vi "DAQ_pp3c_AudioRetrigger.vi"(0 "Daq config In":T6={"Sound AO"="Dev6/ao0", "Shock intesity AO"="Dev6/ao1", "Code_LED DO"="Dev6/port1:2", "Switch DI"="Dev6/port1/line0", "Webcam"="cam9", "Sound AO task"="", "Sound card task"=0, "Shock intensity AO task"="", "Code_LED DO task"="", "Switch DI task"="", "AO <=> Sound card"=FALSE, "Sound card"=0, "sample rate"=100000.0, "Variable shock"=TRUE, "Webcam on"=FALSE, "Waveform memo"={"t0"=timestamp(0 s since 1904-01-01), "dt"=1.0, "Y"=[]}, "Tone trigger"="PFI1", "Master-9 DO"="", "Master-9 DO task"="Dev6/port0/line5:7"} {"sample rate" min=8000.0; "Sound card task" format="%.0x"}, 5 "State In":T1={"Curr  tr"=0, "Curr (ms)"=0, "Cum (ms)"=0, "Run loop diff"=0, "Tone countdown (ms)"=0, "Countdown (ms)"=0, "Curr State"=enum."0 NULL", "Prev State"=enum."1 Habituation", "Rw"=FALSE, "Sw"=FALSE, "Tone\nGate"=FALSE, "Punish"=FALSE, "Current DAQ DO Int"=0, "Current Loaded Trial"={"Trial Type Number"=1, "Trial Type"=enum."GO", "Trial Weight"=100, "Shock (mA)"=0.3, "Duration (ms)"=0.25, "Sound Type"=enum."04 FM Sweep", "Stim P1"=4000.0, "Stim P2"=0.0, "Stim P3"=0.0, "Stim P4"=2000.0, "DAQ Amplitude (V)"=0.25}, "Next Trial (for display purposes)"={"Trial Type Number"=1, "Trial Type"=enum."GO", "Trial Weight"=100, "Shock (mA)"=0.3, "Duration (ms)"=0.25, "Sound Type"=enum."04 FM Sweep", "Stim P1"=4000.0, "Stim P2"=0.0, "Stim P3"=0.0, "Stim P4"=2000.0, "DAQ Amplitude (V)"=0.25}, "Total trials memo"=0, "State start cum memo (ms)"=0, "Last dur jump time memo (ms)"=0, "Last dur shock time memo (ms)"=0, "Tone repeat memo (ms)"=0, "Webcam on"=FALSE, "Webcam recording"=FALSE, "State update flag"=FALSE, "Last loaded shock voltage"=0.0, "Vid upd"=enum."0"} {"Current DAQ DO Int" format="%016b"; "Next Trial (for display purposes)"."DAQ Amplitude (V)" min=0.0 max=5.0 format="%_4g"; "Next Trial (for display purposes)"."Shock (mA)" min=-1.0 max=5.0; "Next Trial (for display purposes)"."Trial Weight" step=1; "Next Trial (for display purposes)"."Duration (ms)" min=0.0 max=1.0; "Next Trial (for display purposes)"."Trial Type Number" min=1 max=256 step=1; "Current Loaded Trial"."DAQ Amplitude (V)" min=0.0 max=5.0 format="%_4g"; "Current Loaded Trial"."Shock (mA)" min=-1.0 max=5.0; "Current Loaded Trial"."Trial Weight" step=1; "Current Loaded Trial"."Duration (ms)" min=0.0 max=1.0; "Current Loaded Trial"."Trial Type Number" min=1 max=256 step=1}, 11 "error in (no error)":errorcluster) -> (4 "Daq config Out":T6={"Sound AO"="Dev6/ao0", "Shock intesity AO"="Dev6/ao1", "Code_LED DO"="Dev6/port1:2", "Switch DI"="Dev6/port1/line0", "Webcam"="cam9", "Sound AO task"="", "Sound card task"=0, "Shock intensity AO task"="", "Code_LED DO task"="", "Switch DI task"="", "AO <=> Sound card"=FALSE, "Sound card"=0, "sample rate"=100000.0, "Variable shock"=TRUE, "Webcam on"=FALSE, "Waveform memo"={"t0"=timestamp(0 s since 1904-01-01), "dt"=1.0, "Y"=[]}, "Tone trigger"="PFI1", "Master-9 DO"="", "Master-9 DO task"="Dev6/port0/line5:7"} {"sample rate" min=8000.0; "Sound card task" format="%.0x"}, 6 "State Out":T1={"Curr  tr"=0, "Curr (ms)"=0, "Cum (ms)"=0, "Run loop diff"=0, "Tone countdown (ms)"=0, "Countdown (ms)"=0, "Curr State"=enum."0 NULL", "Prev State"=enum."1 Habituation", "Rw"=FALSE, "Sw"=FALSE, "Tone\nGate"=FALSE, "Punish"=FALSE, "Current DAQ DO Int"=0, "Current Loaded Trial"={"Trial Type Number"=1, "Trial Type"=enum."GO", "Trial Weight"=100, "Shock (mA)"=0.3, "Duration (ms)"=0.25, "Sound Type"=enum."04 FM Sweep", "Stim P1"=4000.0, "Stim P2"=0.0, "Stim P3"=0.0, "Stim P4"=2000.0, "DAQ Amplitude (V)"=0.25}, "Next Trial (for display purposes)"={"Trial Type Number"=1, "Trial Type"=enum."GO", "Trial Weight"=100, "Shock (mA)"=0.3, "Duration (ms)"=0.25, "Sound Type"=enum."04 FM Sweep", "Stim P1"=4000.0, "Stim P2"=0.0, "Stim P3"=0.0, "Stim P4"=2000.0, "DAQ Amplitude (V)"=0.25}, "Total trials memo"=0, "State start cum memo (ms)"=0, "Last dur jump time memo (ms)"=0, "Last dur shock time memo (ms)"=0, "Tone repeat memo (ms)"=0, "Webcam on"=FALSE, "Webcam recording"=FALSE, "State update flag"=FALSE, "Last loaded shock voltage"=0.0, "Vid upd"=enum."0"} {"Current DAQ DO Int" format="%016b"; "Next Trial (for display purposes)"."DAQ Amplitude (V)" min=0.0 max=5.0 format="%_4g"; "Next Trial (for display purposes)"."Shock (mA)" min=-1.0 max=5.0; "Next Trial (for display purposes)"."Trial Weight" step=1; "Next Trial (for display purposes)"."Duration (ms)" min=0.0 max=1.0; "Next Trial (for display purposes)"."Trial Type Number" min=1 max=256 step=1; "Current Loaded Trial"."DAQ Amplitude (V)" min=0.0 max=5.0 format="%_4g"; "Current Loaded Trial"."Shock (mA)" min=-1.0 max=5.0; "Current Loaded Trial"."Trial Weight" step=1; "Current Loaded Trial"."Duration (ms)" min=0.0 max=1.0; "Current Loaded Trial"."Trial Type Number" min=1 max=256 step=1}, 15 "error out":errorcluster)   [LabVIEW 2013]
uses:
  <vilib>/sound2/lvsound2.llb/Sound Output Write (DBL Single).vi
  <vilib>/sound2/lvsound2.llb/Sound Output Task ID.ctl
  <vilib>/userdefined/High Color/IMAQdx.ctl
  CTL_pp3c_DaqStatus.ctl
  pp3_CTL_State.ctl
  labolabo2/waveforms/WFTypes.ctl
  pp3_CTL_StateInfo.ctl
  pp3_CTL_TrialType.ctl
  pp3_CTL_Trial.ctl
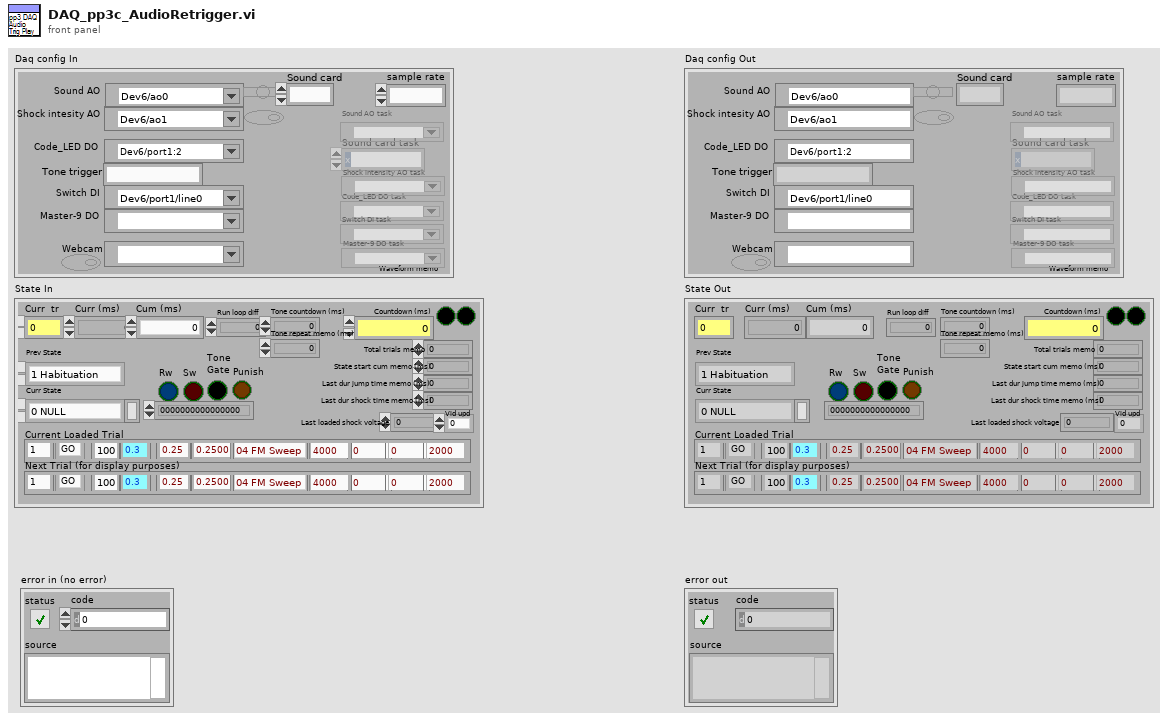
[diagram p1: front panel]
types:
  T1 = typedef "pp3_CTL_StateInfo.ctl" = cluster{"Curr  tr":u16, "Curr (ms)":u32, "Cum (ms)":i64, "Run loop diff":i64, "Tone countdown (ms)":i64, "Countdown (ms)":i64, "Curr State":T2, "Prev State":T2, "Rw":bool, "Sw":bool, "Tone\nGate":bool, "Punish":bool, "Current DAQ DO Int":u16, "Current Loaded Trial":T3, "Next Trial (for display purposes)":T3, "Total trials memo":i64, "State start cum memo (ms)":i64, "Last dur jump time memo (ms)":i64, "Last dur shock time memo (ms)":i64, "Tone repeat memo (ms)":i64, "Webcam on":bool, "Webcam recording":bool, "State update flag":bool, "Last loaded shock voltage":dbl, "Vid upd":enum16{"0", "1", "2", "3", "4", "5", "6", "7", "8", "9"}}
  T2 = typedef "pp3_CTL_State.ctl" = enum8{"0 NULL", "1 Habituation", "2 (Load Trial)", "3 Stay Period", "4 Load Audio/Click Delay", "5 GO Trial", "6 GO Jumped", "7 GO Timeout", "8 NOGO Trial", "9 NOGO Jumped", "10 NOGO Timeout", "11 TEST Trial", "12 TEST Jumped", "13 TEST Timeout", "14 Intertrial Interval", "15 Done"}
  T3 = typedef "pp3_CTL_Trial.ctl" = cluster{"Trial Type Number":i16, "Trial Type":T4, "Trial Weight":u32, "Shock (mA)":dbl, "Duration (ms)":dbl, "Sound Type":T5, "Stim P1":dbl, "Stim P2":dbl, "Stim P3":dbl, "Stim P4":dbl, "DAQ Amplitude (V)":dbl}
  T4 = typedef "pp3_CTL_TrialType.ctl" = enum16{"OFF", "GO", "NOGO", "TEST"}
  T5 = typedef "WFTypes.ctl" = enum16{"00 NULL", "01 DC", "02 Noise", "03 Pure Tone", "04 FM Sweep"}
  T6 = typedef "CTL_pp3c_DaqStatus.ctl" = cluster{"Sound AO":tag, "Shock intesity AO":tag, "Code_LED DO":tag, "Switch DI":tag, "Webcam":T7, "Sound AO task":refnum<k21>, "Sound card task":T8, "Shock intensity AO task":refnum<k21>, "Code_LED DO task":refnum<k21>, "Switch DI task":refnum<k21>, "AO <=> Sound card":bool, "Sound card":u32, "sample rate":dbl, "Variable shock":bool, "Webcam on":bool, "Waveform memo":waveform(dbl), "Tone trigger":string, "Master-9 DO":tag, "Master-9 DO task":refnum<k21>}
  T7 = typedef "IMAQdx.ctl" = refnum<k21>
  T8 = typedef "Sound Output Task ID.ctl" = u32
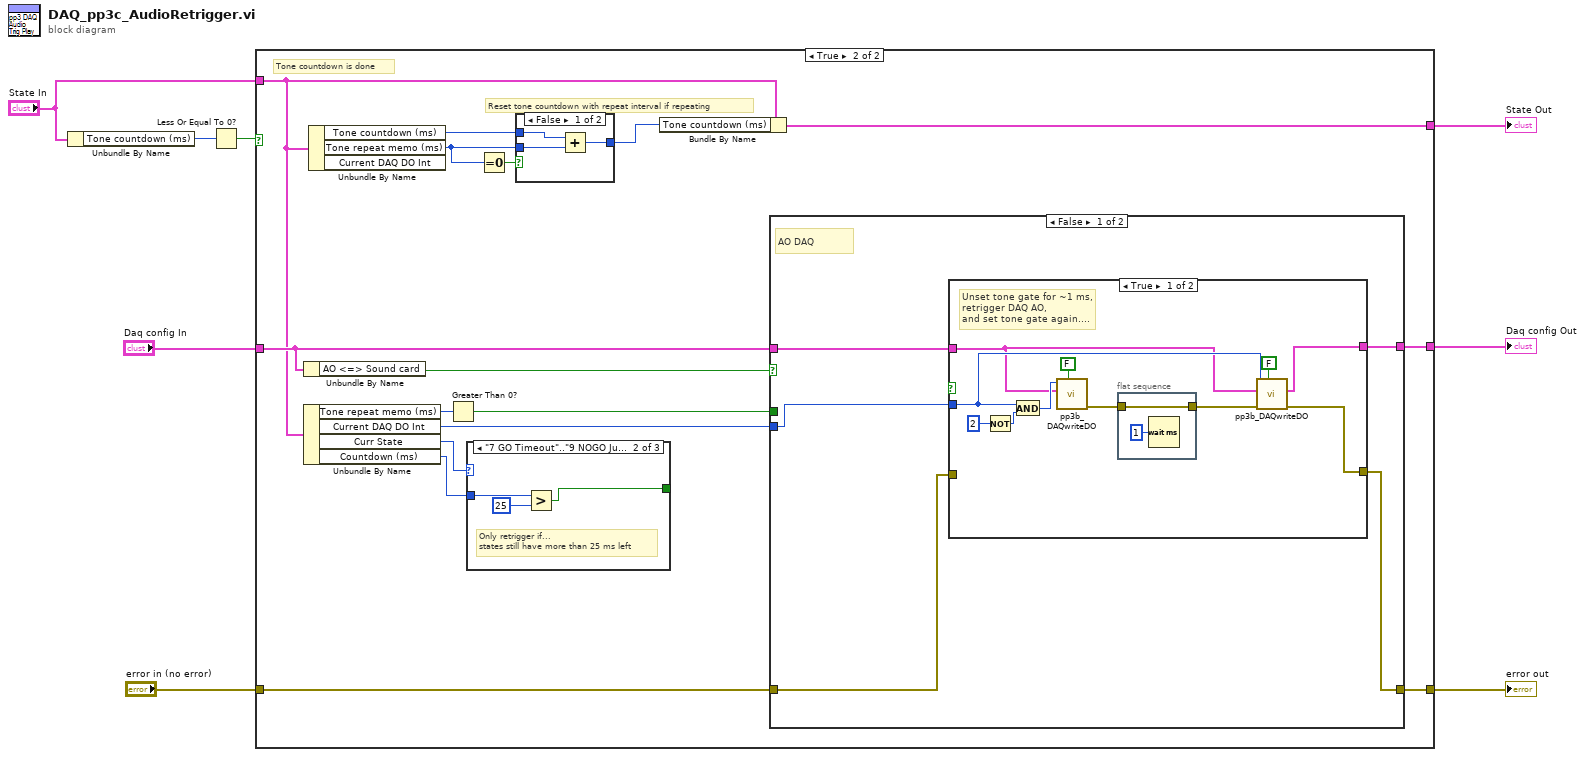
[diagram p0: block diagram]
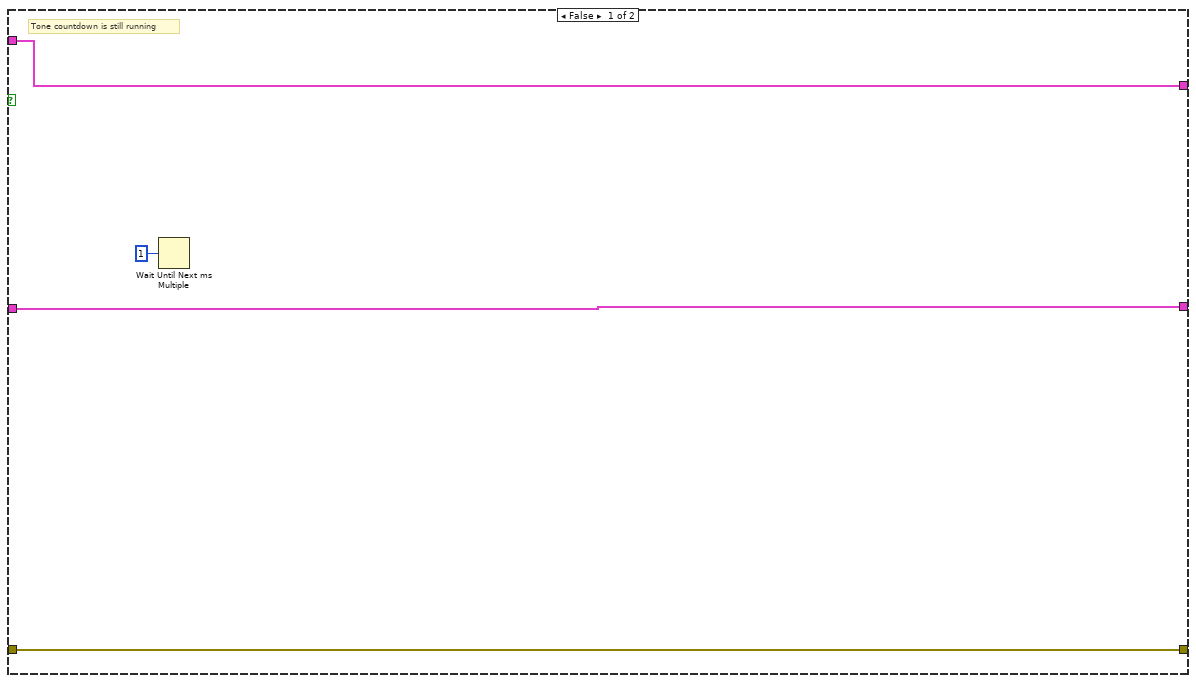
[diagram p2: hidden frame]
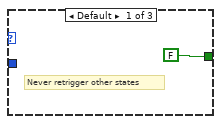
[diagram p3: hidden frame]
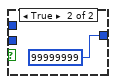
[diagram p5: hidden frame]
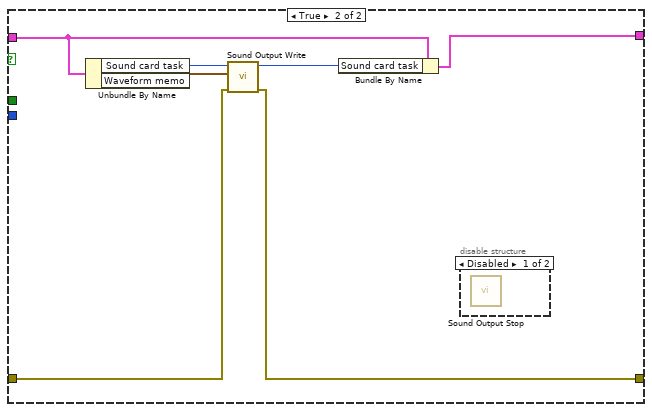
[diagram p7: hidden frame]
diagram:
  n1 = Unbundle By Name("State In") -> ("Tone countdown (ms)"=w4:i64)
  n2 = Less Or Equal To 0?(x=w4) -> (x <= 0?=w1:bool)
  n3 = case shown="True" w1 {
    tunnel: "Daq config In" -> [w12 w25]
    tunnel: [w12 w24] -> w7
    tunnel: "error in (no error)" -> [w11 w27]
    tunnel: [w11 w26] -> w5
    tunnel: "State In" -> [w9 w15]
    tunnel: [w9 w23] -> w2
    frame False {
      # "Tone countdown is still running"
      n4 = Wait Until Next ms Multiple(millisecond multiple=u32 1) -> ()  [unwired: 1 out]
    }
    frame True {
      # "Tone countdown is done"
      # "Reset tone countdown with repeat interval if repeating"
      n5 = Unbundle By Name(w25) -> ("AO <=> Sound card"=w28:bool)
      n6 = Unbundle By Name(w15) -> ("Tone repeat memo (ms)"=w18:i64, "Current DAQ DO Int"=w16:u16, "Curr State"=w14:T2, "Countdown (ms)"=w13:i64)
      n7 = Unbundle By Name(w15) -> ("Tone countdown (ms)"=w20:i64, "Tone repeat memo (ms)"=w21:i64)  [unwired: 1 out]
      n8 = Greater Than 0?(x=w18) -> (x > 0?=w17:bool)
      n9 = case shown="\"7 GO Timeout\"..\"9 NOGO Jumped\", \"11 TEST Trial\"" w14 {
        tunnel: [FALSE w30 _] -> _
        tunnel: w13 -> [_ w31 _]
        frame Default {
          # "Never retrigger other states"
        }
        frame "7 GO Timeout".."9 NOGO Jumped", "11 TEST Trial" {
          # "Only retrigger if...\nstates still have more than 25 ms left"
          n10 = Greater?(x=w31, y=i64 25) -> (0:w30:bool)
        }
        frame "5 GO Trial" {
          # "GO Trial always retriggered\neven when <25 ms left,\nsince end leads to\ntone cont/shock (miss)"
        }
      }
      n11 = Equal To 0?(x=w21) -> (x = 0?=w22:bool)
      n12 = case shown="False" w22 {
        tunnel: w21 -> [w34 _]
        tunnel: w20 -> [w35 _]
        tunnel: [w33 i64 99999999] -> w19
        frame False {
          n13 = Add(x=w35, y=w34) -> (x+y=w33:i64)
        }
        frame True {
        }
      }
      n14 = Bundle By Name(cluster=w15, "Tone countdown (ms)"=w19) -> (w23:T1)
      n15 = case shown="False" w28 {
        tunnel: w27 -> [w38 w62]
        tunnel: [w41 w61] -> w26
        tunnel: w25 -> [w40 w59]
        tunnel: [w39 w60] -> w24
        tunnel: w17 -> [_ _]
        tunnel: w16 -> [w37 _]
        frame False {
          # "AO DAQ"
          n16 = case shown="True" {
            selector: _ -> [_ _]
            tunnel: w38 -> [_ w54]
            tunnel: [w48 w54] -> w41
            tunnel: w40 -> [w43 w55]
            tunnel: [w43 w55] -> w39
            tunnel: w37 -> [w46 _]
            frame True {
              # "Unset tone gate for ~1 ms,\nretrigger DAQ AO,\nand set tone gate again...."
              n17 = Not(x=u16 2) -> (.not. x?=w50:u16)
              n18 = And(x=w46, y=w50) -> (x .and. y?=w49:u16)
              n19 = call "pp3b_DAQwriteDO.vi"("Reset to zero"=FALSE, "Daq config"=w43, "DAQ Digital In"=w49) -> ("error out"=w47:errorcluster)  [unwired: 8 in]
              n20 = flat-sequence {
                tunnel: [w52] -> w42
                tunnel: w47 -> [w52]
                frame #0 {
                  n21 = Wait (ms)(milliseconds to wait=u32 1) -> ()  [unwired: 1 out]
                }
              }
              n22 = call "pp3b_DAQwriteDO.vi"("Reset to zero"=FALSE, "error in (no error)"=w42, "Daq config"=w43, "DAQ Digital In"=w46) -> ("error out"=w48:errorcluster)  [unwired: 7 in]
            }
            frame False {
            }
          }
        }
        frame True {
          n23 = Unbundle By Name(w59) -> ("Sound card task"=w58:T8, "Waveform memo"=w57:waveform(dbl))
          n24 = call-poly <vilib>:"Sound Output Write.vi"("error in (no error)"=w62, "data"=w57, "task ID"=w58) -> ("error out"=w61:errorcluster, "task ID out"=w56:T8)  [unwired: 7 in]
          n25 = Bundle By Name(cluster=w59, "Sound card task"=w56) -> (w60:T6)
          n26 = disable-structure shown="Disabled" {
            frame Disabled {
              n27 = call <vilib>:"Sound Output Stop.vi"() -> ()  [unwired: 10 in, 2 out]
            }
            frame Enabled {
            }
          }
        }
      }
    }
  }
  "Daq config Out" <- w7
  "error out" <- w5
  "State Out" <- w2
